vi "SetVoltRange(General).vi"(8 "Error In":errorcluster, 10 "Range":string(combo)="AUTO", 11 "VISA resource name":refnum<visa-resource-name>) -> (0 "Error Out":errorcluster, 3 "VISA resource name out":refnum<visa-resource-name>)   [LabVIEW 2013]
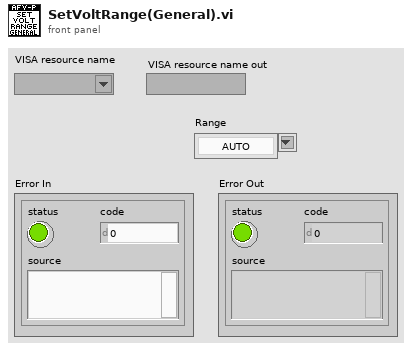
[diagram p1: front panel]
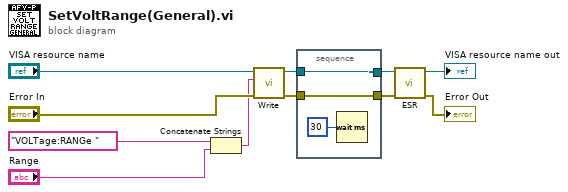
[diagram p0: block diagram]
diagram:
  n1 = Concatenate Strings("VOLTage:RANGe " ("Write Buffer"), "Range") -> (w8:string)
  n2 = call "Write.vi"("Error In"="Error In", "Write Buffer"=w8, "VISA resource name"="VISA resource name") -> ("Error Out"=w3:errorcluster, "VISA resource name out"=w4:refnum<visa-resource-name>)  [unwired: 7 in]
  n3 = stacked-sequence {
    tunnel: [w13] -> w6
    tunnel: w4 -> [w13]
    tunnel: [w12] -> w5
    tunnel: w3 -> [w12]
    frame #0 {
      n4 = Wait (ms)(milliseconds to wait=u32 30) -> ()  [unwired: 1 out]
    }
  }
  n5 = call "ESR.vi"("Error In"=w5, "VISA resource name"=w6) -> ("Error Out"=→"Error Out":errorcluster, "VISA resource name out"=→"VISA resource name out":refnum<visa-resource-name>)  [unwired: 8 in]
